vi "add_analysis_data.vi"(8 "error in (no error)":errorcluster, 10 "data array":string[](array[string]), 11 "Analysis in":refnum<class "Analysis.lvclass">) -> (0 "error out":errorcluster, 2 "data array out":string[](array[string]), 3 "Analysis out":refnum<class "Analysis.lvclass">)   [LabVIEW 2017]
doc: "input is the data array from the text file.\nThe VI searches for the analysis data and writes the data into the AnalysisObject"
uses:
  MSControl/Classes/Analysis/Analysis.lvclass
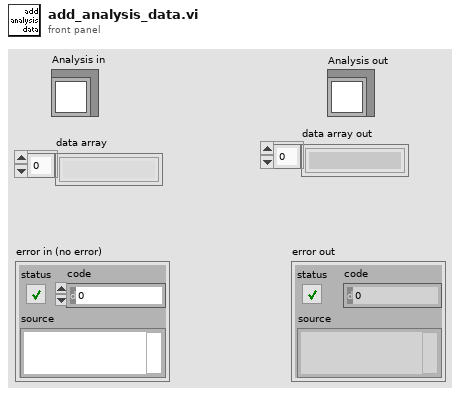
[diagram p1: front panel]
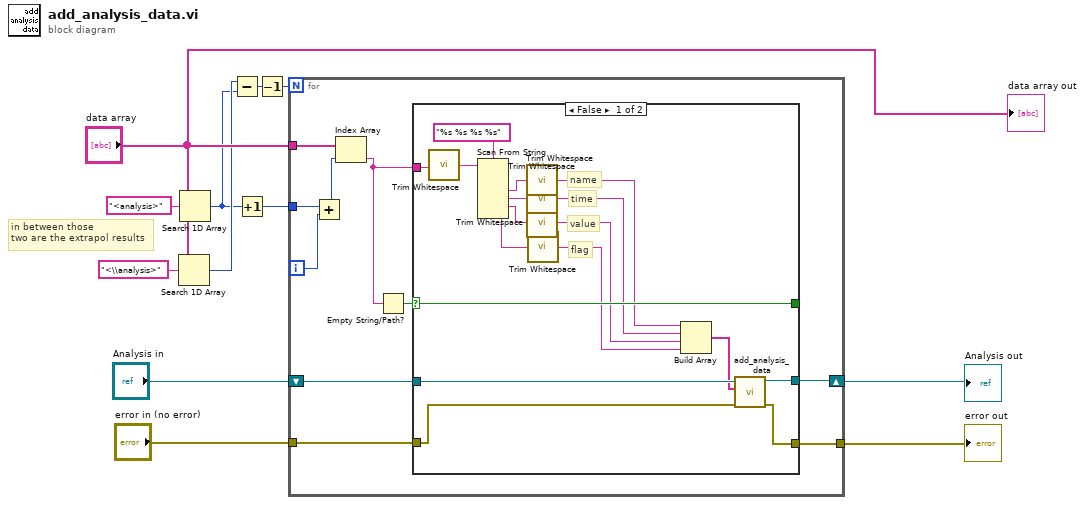
[diagram p0: block diagram]
diagram:
  # "in between those\ntwo are the extrapol results"
  n1 = Search 1D Array(1D array="data array", element="<\\analysis>") -> (index of element=w9:i32)  [unwired: 1 in]
  n2 = Search 1D Array(1D array="data array", element="<analysis>") -> (index of element=w7:i32)  [unwired: 1 in]
  n3 = Subtract(x=w9, y=w7) -> (x-y=w6:i32)
  n4 = Increment(x=w7) -> (x+1=w8:i32)
  n5 = Decrement(x=w6) -> (x-1=w5:i32)
  n6 = for {
    N: w5 -> [_]
    tunnel: "data array" -> [w22]
    tunnel: w8 -> [w21]
    tunnel: "error in (no error)" -> [w15]
    shift-right: [w14] -> w1
    shift-left: "Analysis in" -> [w16]
    tunnel: [w13] -> w2
    i -> [w20]
    n7 = Add(x=w21, y=w20) -> (x+y=w19:i32)
    n8 = Index Array(array=w22, index=w19) -> (element=w18:string)
    n9 = Empty String/Path?(string/path=w18) -> (empty?=w17:bool)
    n10 = case shown="False" w17 {
      selector: w17 -> [w36 w42]
      tunnel: w18 -> [w37 _]
      tunnel: [w36 w42] -> _
      tunnel: w16 -> [w32 w41]
      tunnel: w15 -> [w29 w40]
      tunnel: [w31 w41] -> w14
      tunnel: [w28 w40] -> w13
      frame False {
        # "flag"
        # "value"
        # "time"
        # "name"
        n11 = call <vilib>:"Trim Whitespace.vi"("string"=w37) -> ("trimmed string"=w39:string)  [unwired: 1 in]
        n12 = Scan From String(format string="%s %s %s %s", input string=w39) -> (output 1=w35:string, output 2=w27:string, output 3=w26:string, output 4=w23:string)  [unwired: 6 in, 3 out]
        n13 = call <vilib>:"Trim Whitespace.vi"("string"=w35) -> ("trimmed string"=w34:string)  [unwired: 1 in]
        n14 = call <vilib>:"Trim Whitespace.vi"("string"=w27) -> ("trimmed string"=w33:string)  [unwired: 1 in]
        n15 = call <vilib>:"Trim Whitespace.vi"("string"=w26) -> ("trimmed string"=w25:string)  [unwired: 1 in]
        n16 = call <vilib>:"Trim Whitespace.vi"("string"=w23) -> ("trimmed string"=w24:string)  [unwired: 1 in]
        n17 = Build Array(w34, w33, w25, w24) -> (w30:string[])
        n18 = call-dynamic "add_analysis_data.vi"("error in (no error)"=w29, "single analysis data"=w30, "Analysis in"=w32) -> ("error out"=w28:errorcluster, "Analysis out"=w31:refnum<class "Analysis.lvclass">)  [unwired: 7 in]
      }
      frame True {
      }
    }
  }
  "Analysis out" <- w1
  "error out" <- w2
  "data array out" <- "data array"
